vi "set EPA FileName.vi"(10 "File Name EPA":string, 11 "FileNameInput References":T1) -> ()   [LabVIEW 2020, in "Linearisierung v2.lvlib" / "SpanEinstellungen.lvlib"]
uses:
  SpanEinstellungen.lvlib
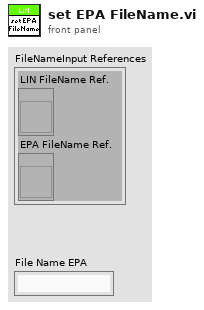
[diagram p1: front panel]
types:
  T1 = cluster{"LIN FileName Ref.":refnum<vi>, "EPA FileName Ref.":refnum<vi>}
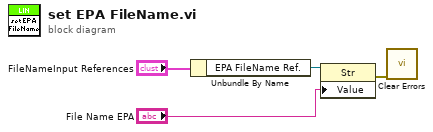
[diagram p0: block diagram]
diagram:
  n1 = Unbundle By Name("FileNameInput References") -> ("EPA FileName Ref."=w3:refnum<vi>)
  n2 = property class="Str"(reference=w3, "Value"="File Name EPA") -> (error out=w1:errorcluster)  [unwired: 1 in, 1 out]
  n3 = call <vilib>:"Clear Errors.vi"("error in (no error)"=w1) -> ()  [unwired: 5 in, 2 out]
